vi "Send RECIBIR_PARAMETROS.vi"(7 "Message Priority (Normal)":T2=enum."Normal", 8 "error in (no error)":errorcluster, 10 "Parámetros":T1={"signal type"=enum."Sine Wave", "amplitude"=1.0, "frequency"=10.0} {"frequency" format="%0.2p"; "amplitude" format="%0.2p"}, 11 "Message Enqueuer":refnum<class "Message Enqueuer.lvclass">) -> (0 "error out":errorcluster, 3 "Message Enqueuer out":refnum<class "Message Enqueuer.lvclass">)   [LabVIEW 2019, in "GRAFICAR_SEÑAL_ACTUALIZABLE.lvlib" / "RECIBIR_PARAMETROS Msg.lvclass"]
doc: "This VI sends the message to an actor."
uses:
  RECIBIR_PARAMETROS Msg.lvclass
  <vilib>/ActorFramework/Message Enqueuer/Message Enqueuer.lvclass
  <vilib>/ActorFramework/Message Enqueuer/Message Priority.ctl
  C:/Program Files (x86)/National Instruments/LabVIEW 2019/vi.lib/ActorFramework/Message/Message.lvclass
  RECIBIR_PARAMETROS Msg.lvclass/RECIBIR_PARAMETROS Msg.ctl
  <vilib>/ActorFramework/Message Enqueuer/Message Enqueuer.lvclass/Message Enqueuer.ctl
  <vilib>/ActorFramework/Message Priority Queue/Priority Enqueue.vi
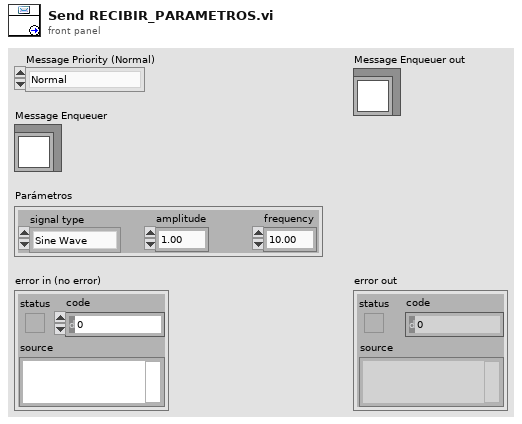
[diagram p1: front panel]
types:
  T1 = cluster{"signal type":enum16{"Sine Wave", "Triangle Wave", "Square Wave", "Sawtooth Wave"}, "amplitude":dbl, "frequency":dbl}
  T2 = typedef "Actor Framework.lvlib/Message Enqueuer.lvclass/Message Priority.ctl" = enum16{"Low", "Normal", "High"}
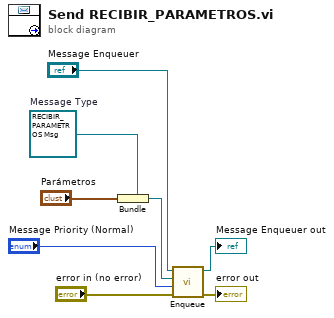
[diagram p0: block diagram]
diagram:
  w5 = refnum<class "RECIBIR_PARAMETROS Msg.lvclass"> refnum  # Message Type
  n1 = Bundle(cluster=w5, "Parámetros") -> (w4:refnum<class "RECIBIR_PARAMETROS Msg.lvclass">)
  n2 = call <vilib>:"Enqueue.vi"("error in (no error)"="error in (no error)", "Message Priority (Normal)"="Message Priority (Normal)", "Message"=w4, "Message Enqueuer in"="Message Enqueuer") -> ("error out"=→"error out":errorcluster, "Message Enqueuer out"=→"Message Enqueuer out":refnum<class "Message Enqueuer.lvclass">)  [unwired: 6 in]
